vi "Get Icon Source Path INI.vi"(8 "error in":errorcluster, 11 "config.ini path":path) -> (0 "error out":errorcluster, 2 "Icon source dir":path, 3 "config.ini path dup":path)   [LabVIEW 2012]
uses:
  INI_source.ctl
  <userlib>/_OpenG.lib/file/file.llb/File Exists - Scalar__ogtk.vi
  <userlib>/_OpenG.lib/file/file.llb/Build Path - Traditional__ogtk.vi
  <userlib>/_OpenG.lib/file/file.llb/Strip Path - Traditional__ogtk.vi
  <vilib>/Utility/config.llb/NI_LVConfig.lvlib
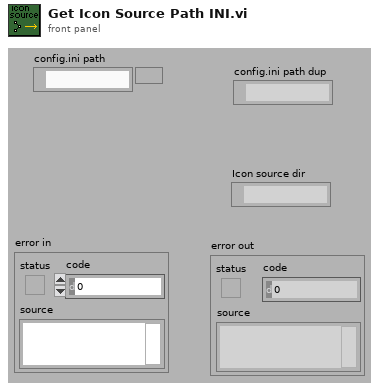
[diagram p1: front panel]
types:
  T1 = typedef "INI_source.ctl" = cluster{"Icon source":path}
  T2 = typedef "NI_LVConfig.lvlib/Config Data RefNum.ctl" = refnum<k1>
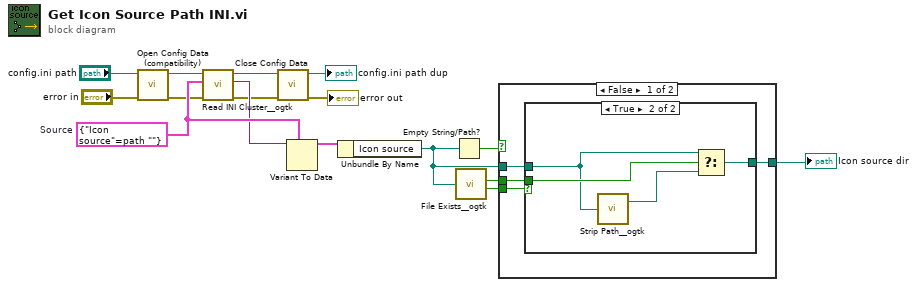
[diagram p0: block diagram]
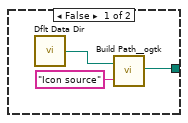
[diagram p2: hidden frame]
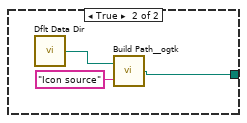
[diagram p3: hidden frame]
diagram:
  w16 = T1 {"Icon source"=path ""}  # Source
  n1 = call <vilib>:"Open Config Data (compatibility).vi"("error in (no error)"="error in", "configuration file path"="config.ini path") -> ("error out"=w2:errorcluster, "refnum"=w1:T2)  [unwired: 7 in, 1 out]
  n2 = call <userlib>:"Read INI Cluster__ogtk.vi"("error in (no error)"=w2, "INI Fomatted Cluster Type"=w16, "refnum"=w1) -> ("error out"=w8:errorcluster, "INI Fomatted Cluster"=w9:variant, "dup refnum"=w7:T2)  [unwired: 6 out]
  n3 = call <vilib>:"Close Config Data.vi"("error in (no error)"=w8, "refnum"=w7) -> ("error out"=→"error out":errorcluster, "file path"=→"config.ini path dup":path)  [unwired: 1 in, 7 out]
  n4 = Variant To Data(type=w16, Variant=w9) -> (data=w10:T1)  [unwired: 1 in, 1 out]
  n5 = Unbundle By Name(w10) -> ("Icon source"=w14:path)
  n6 = Empty String/Path?(string/path=w14) -> (empty?=w11:bool)
  n7 = call-poly <userlib>:"File Exists__ogtk.vi"("file path"=w14) -> ("is directory"=w12:bool, "exists"=w13:bool)  [unwired: 6 in]
  n8 = case shown="False" w11 {
    tunnel: [w20 w28] -> w15
    tunnel: w12 -> [w17 _]
    tunnel: w13 -> [w18 _]
    tunnel: w14 -> [w19 _]
    frame False {
      n9 = case shown="True" w18 {
        tunnel: [w21 w27] -> w20
        tunnel: w19 -> [_ w25]
        tunnel: w17 -> [_ w26]
        frame False {
          n10 = call <vilib>:"Dflt Data Dir.vi"() -> ("App:Default Data Directory"=w23:path)
          n11 = call-poly <userlib>:"Build Path__ogtk.vi"("name or relative path"="Icon source", "base path"=w23) -> ("appended path"=w21:path)
        }
        frame True {
          n12 = call-poly <userlib>:"Strip Path__ogtk.vi"("path"=w25) -> ("stripped path"=w24:path)  [unwired: 1 out]
          n13 = Select(t=w25, s=w26, f=w24) -> (s? t:f=w27:path)
        }
      }
    }
    frame True {
      n14 = call <vilib>:"Dflt Data Dir.vi"() -> ("App:Default Data Directory"=w30:path)
      n15 = call-poly <userlib>:"Build Path__ogtk.vi"("name or relative path"="Icon source", "base path"=w30) -> ("appended path"=w28:path)
    }
  }
  "Icon source dir" <- w15
